vi "Watch Dog Write.vi"(1 "Set D.In":string[](array[string])=["1"]) -> (0 "Set D.In 2":string[](array[string]))   [LabVIEW 2015]
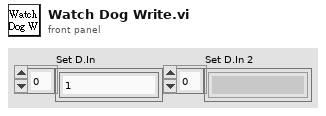
[diagram p1: front panel]
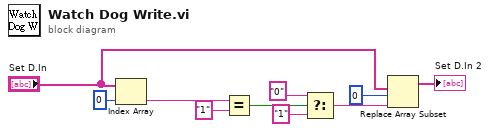
[diagram p0: block diagram]
diagram:
  n1 = Index Array(array="Set D.In", index=0) -> (element=w8:string)
  n2 = Equal?(x=w8, y="1") -> (x = y?=w10:bool)
  n3 = Select(t="0" ("y"), s=w10, f="1") -> (s? t:f=w4:string)
  n4 = Replace Array Subset(array="Set D.In", new element=w4, index=0) -> (→"Set D.In 2":string[])
